vi "Increment Score.vi"(10 "Score ref in":refnum<vi>) -> (0 "error out":errorcluster)   [LabVIEW 2024, in "Game Board.lvclass"]
doc: "MIT Licence\nCopyright (c) 2024 David Grollier"
uses:
  Game Board.lvclass
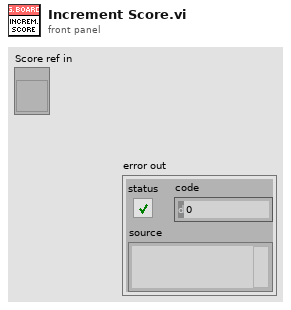
[diagram p1: front panel]
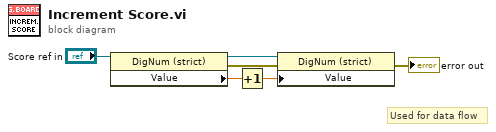
[diagram p0: block diagram]
diagram:
  # "Used for data flow"
  n1 = property class="DigNum (strict)"(reference="Score ref in") -> (reference out=w3:refnum<vi>, error out=w4:errorcluster, "Value"=w5:dbl)  [unwired: 1 in]
  n2 = Increment(x=w5) -> (x+1=w6:dbl)
  n3 = property class="DigNum (strict)"(reference=w3, error in=w4, "Value"=w6) -> (error out=→"error out":errorcluster)  [unwired: 1 out]
